vi "Data.Engine.Initialize.vi"(8 "error in":errorcluster, 9 "Compiled.InlineAsync.Settings":variant, 10 "PluginAPIs":T1=refnum) -> (0 "error out":errorcluster, 2 "Data Access Engine":refnum<class "Plugin Data Access Engine.lvclass">)   [LabVIEW 2023, in "Plugin Data Access Engine.lvlib" / "Plugin Data Access Engine.lvclass"]
uses:
  Plugin Data Access Engine.lvclass
  Plugin Data Access Engine.lvclass/Plugin Data Access Engine.ctl
  <vilib>/NI VeriStand/Custom Device API/Data Reference.ctl
  <vilib>/NI VeriStand/Custom Device API/Block Data Reference.ctl
  Access Type Classes/Read/Read.lvclass
  Access Type Classes/Write/Write.lvclass
  Access Type Classes/ReadWrite/ReadWrite.lvclass
  <userlib>/PluginCore_v1.lvlibp/iPluginAPIs/iPluginAPIs.lvclass
  _PluginCore/Types/Plugin API.ctl
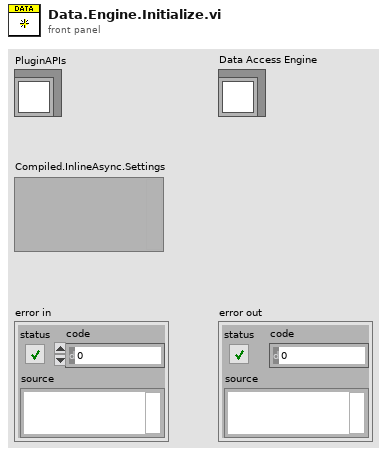
[diagram p1: front panel]
types:
  T1 = typedef "Plugin API.ctl" = refnum<class "iPluginAPIs.lvclass">
  T2 = typedef "Custom Device API.lvlib/Block Data Reference.ctl" = cluster{"Data Reference":T3, "Offset":u64, "Length":u64}
  T3 = typedef "Custom Device API.lvlib/Data Reference.ctl" = i32
  T4 = cluster{"Read":cluster{"Refs":T2[], "Values":dbl[]}[], "Write":cluster{"Refs":T2[], "Values":dbl[]}[], "ReadWrite":cluster{"Refs":T3[], "Values":dbl[], "Reset Values":dbl[]}[], "LUT":variant}
  T5 = cluster{"Refs":T3[], "Values":dbl[], "Reset Values":dbl[]}[]
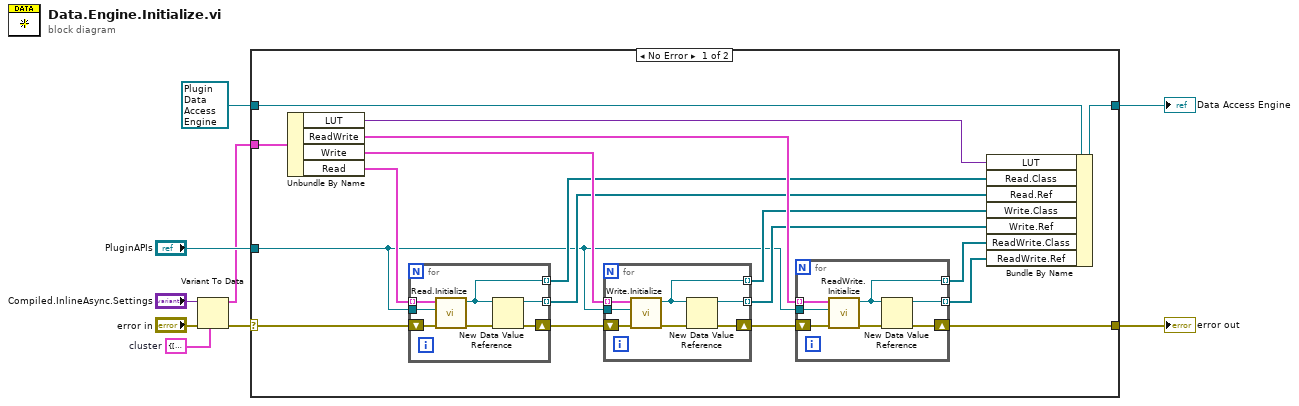
[diagram p0: block diagram]
diagram:
  w8 = T4 {"Read"=[], "Write"=[], "ReadWrite"=[], "LUT"=variant}  # cluster
  n1 = Variant To Data(error in="error in", type=w8, Variant="Compiled.InlineAsync.Settings") -> (data=w3:T4, error out=w2:errorcluster)
  n2 = case shown="No Error" w2 {
    selector: w2 -> [w26 w50]
    tunnel: [w23 w50] -> w6
    tunnel: [w17 w49] -> w7
    tunnel: refnum<class "Plugin Data Access Engine.lvclass"> refnum ("Data Access API.lvlib:Data Access API.lvclass") -> [w12 w49]
    tunnel: w3 -> [w13 _]
    tunnel: "PluginAPIs" -> [w10 _]
    frame No Error {
      n3 = Unbundle By Name(w13) -> ("LUT"=w11:variant, "ReadWrite"=w21:T5, "Write"=w22:cluster{"Refs":T2[], "Values":dbl[]}[], "Read"=w27:cluster{"Refs":T2[], "Values":dbl[]}[])
      n4 = for {
        tunnel: w27 -> [w48] mode=indexing
        shift-right: [w45] -> w25
        shift-left: w26 -> [w47]
        tunnel: [w44] -> w18 mode=indexing
        tunnel: [w43] -> w14 mode=indexing
        tunnel: w10 -> [w42]
        n5 = call "Read.Initialize.vi"("error in"=w47, "PluginAPIs"=w42, "Settings"=w48) -> ("error out"=w46:errorcluster, "Read out"=w44:refnum<class "Read.lvclass">)  [unwired: 7 in]
        n6 = New Data Value Reference(data value=w44, error in=w46) -> (data value reference=w43:refnum<data-value>, error out=w45:errorcluster)
      }
      n7 = for {
        tunnel: w22 -> [w41] mode=indexing
        shift-right: [w37] -> w24
        shift-left: w25 -> [w40]
        tunnel: [w39] -> w19 mode=indexing
        tunnel: [w36] -> w15 mode=indexing
        tunnel: w10 -> [w35]
        n8 = call "Write.Initialize.vi"("error in"=w40, "PluginAPIs"=w35, "Settings"=w41) -> ("error out"=w38:errorcluster, "Write out"=w39:refnum<class "Write.lvclass">)  [unwired: 7 in]
        n9 = New Data Value Reference(data value=w39, error in=w38) -> (data value reference=w36:refnum<data-value>, error out=w37:errorcluster)
      }
      n10 = for {
        tunnel: w21 -> [w33] mode=indexing
        shift-right: [w31] -> w23
        shift-left: w24 -> [w34]
        tunnel: [w30] -> w20 mode=indexing
        tunnel: [w29] -> w16 mode=indexing
        tunnel: w10 -> [w28]
        n11 = call "ReadWrite.Initialize.vi"("error in"=w34, "PluginAPIs"=w28, "Settings"=w33) -> ("error out"=w32:errorcluster, "ReadWrite out"=w30:refnum<class "ReadWrite.lvclass">)  [unwired: 7 in]
        n12 = New Data Value Reference(data value=w30, error in=w32) -> (data value reference=w29:refnum<data-value>, error out=w31:errorcluster)
      }
      n13 = Bundle By Name(cluster=w12, "LUT"=w11, "Read.Class"=w18, "Read.Ref"=w14, "Write.Class"=w19, "Write.Ref"=w15, "ReadWrite.Class"=w20, "ReadWrite.Ref"=w16) -> (w17:refnum<class "Plugin Data Access Engine.lvclass">)
    }
    frame Error {
    }
  }
  "error out" <- w6
  "Data Access Engine" <- w7
